vi "Write Averaging time.vi"(8 "error in (no error)":errorcluster, 10 "Averaging time":dbl, 11 "Red Pitaya in":refnum<class "Red Pitaya.lvclass">) -> (0 "error out":errorcluster, 3 "Red Pitaya out":refnum<class "Red Pitaya.lvclass">)   [LabVIEW 2015, in "Red Pitaya.lvclass"]
uses:
  Red Pitaya.lvclass
  Red Pitaya.lvclass/Red Pitaya.ctl
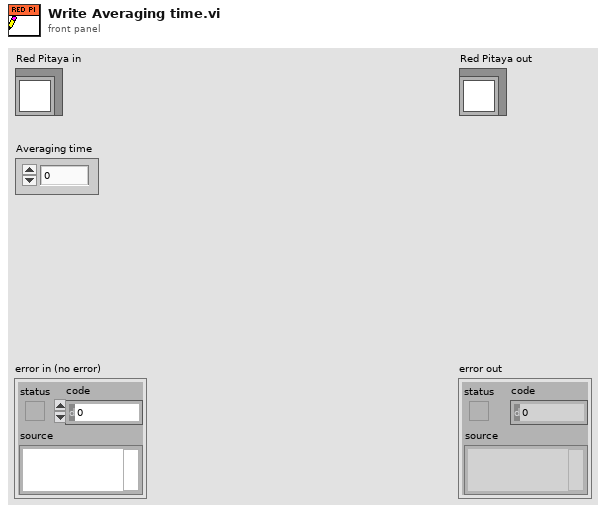
[diagram p1: front panel]
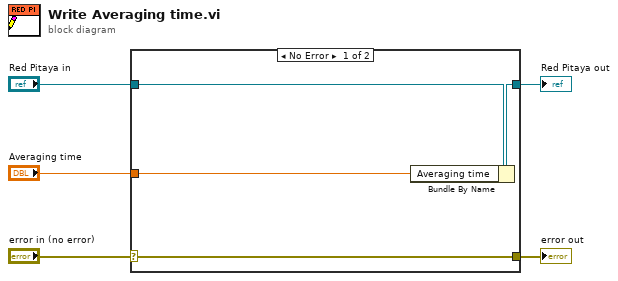
[diagram p0: block diagram]
diagram:
  n1 = case shown="No Error" "error in (no error)" {
    selector: "error in (no error)" -> [w9 w10]
    tunnel: [w9 w10] -> w4
    tunnel: [w7 w11] -> w2
    tunnel: "Red Pitaya in" -> [w8 w11]
    tunnel: "Averaging time" -> [w6 _]
    frame No Error {
      n2 = Bundle By Name(cluster=w8, "Averaging time"=w6) -> (w7:refnum<class "Red Pitaya.lvclass">)
    }
    frame Error {
    }
  }
  "error out" <- w4
  "Red Pitaya out" <- w2
